vi "TxtToExcel v4.vi"() -> ()   [LabVIEW 2016]
panel:
  out "output array":string[][](array[string])
  out "error out":errorcluster
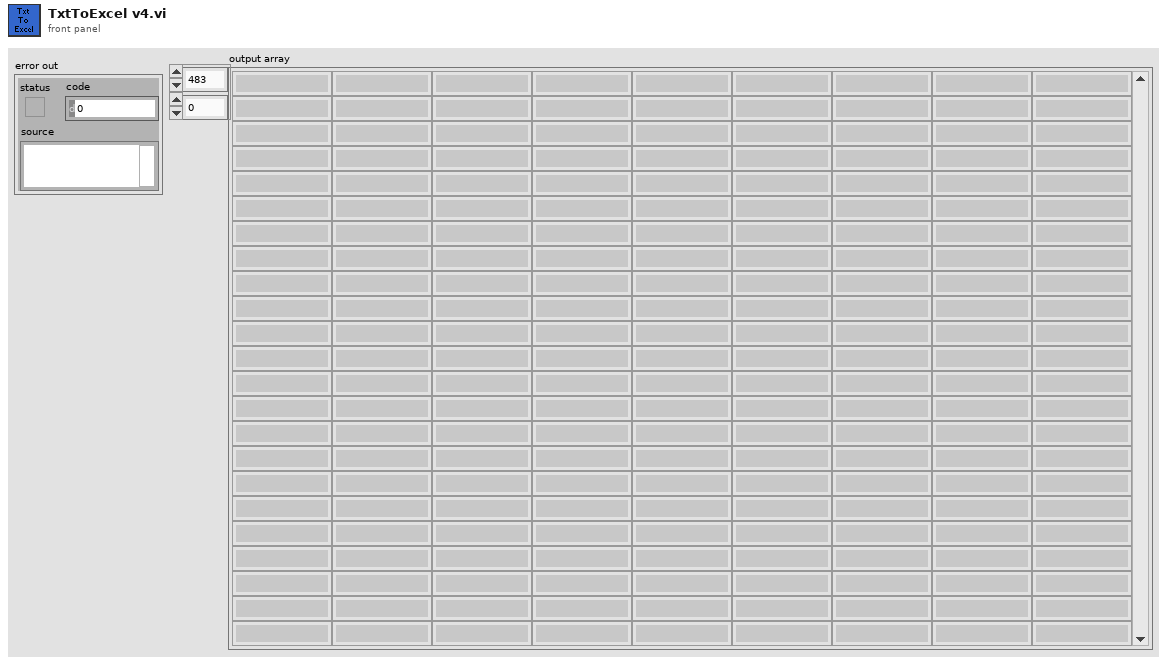
[diagram p1: front panel]
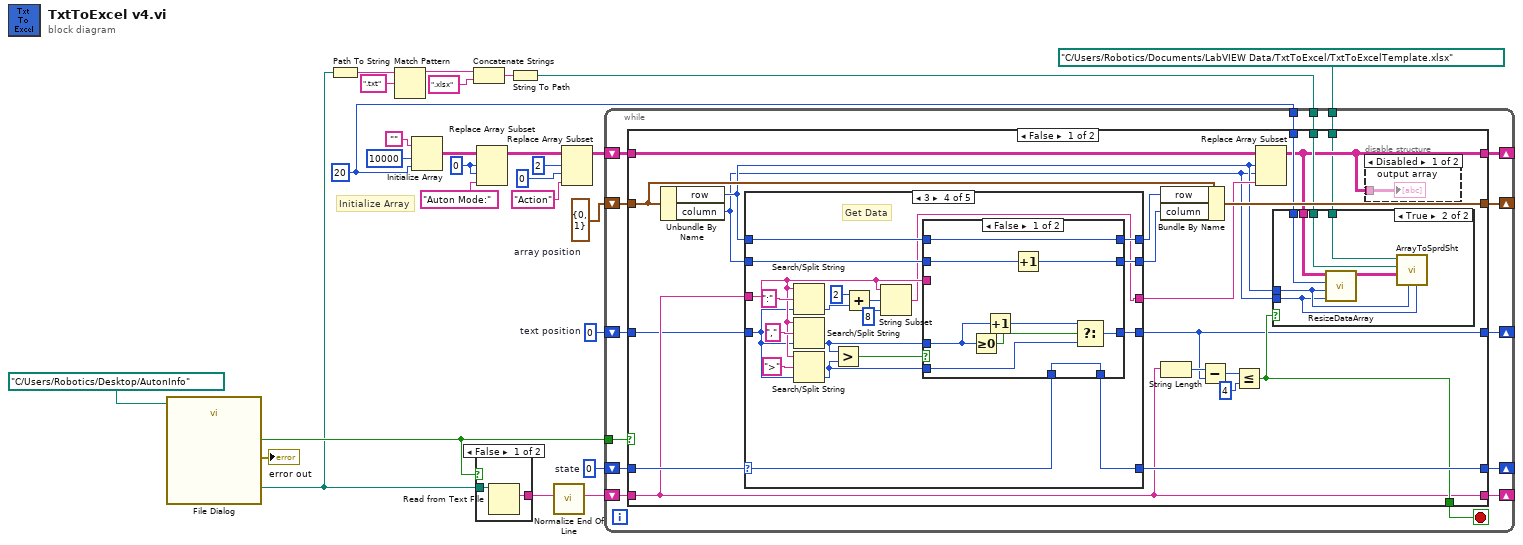
[diagram p0: block diagram]
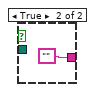
[diagram p2: hidden frame]
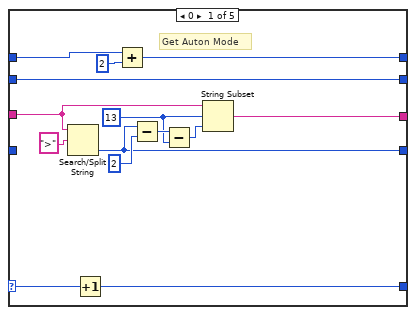
[diagram p5: hidden frame]
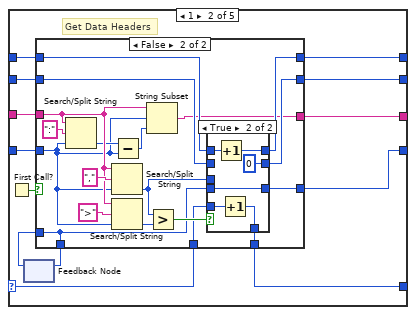
[diagram p6: hidden frame]
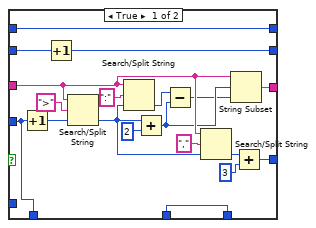
[diagram p7: hidden frame]
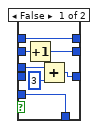
[diagram p8: hidden frame]
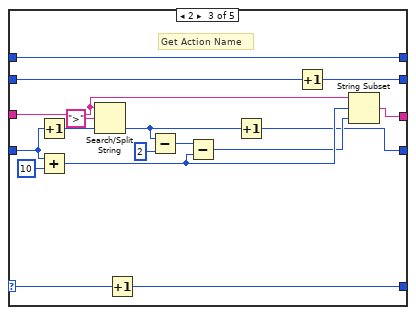
[diagram p9: hidden frame]
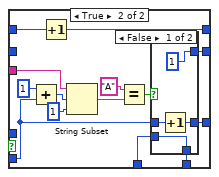
[diagram p10: hidden frame]
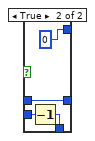
[diagram p11: hidden frame]
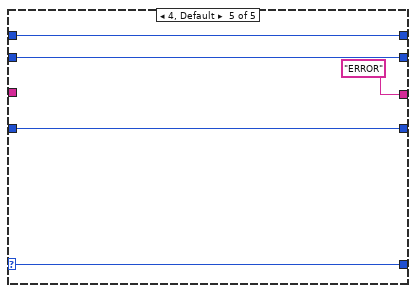
[diagram p12: hidden frame]
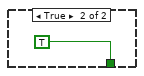
[diagram p13: hidden frame]
diagram:
  w2 = 0  # text position
  w17 = 0 ("index (row)")
  w19 = cluster{"row":i32, "column":i32} {"row"=0, "column"=1}  # array position
  w3 = 20 ("Column Max")
  w24 = 0  # state
  # "Initialize Array"
  n1 = call "File Dialog"("start path"=path "C:/Users/Robotics/Desktop/AutonInfo") -> ("selected path"=w10:path, "cancelled"=w25:bool, "error out"=→"error out":errorcluster)  [unwired: 11 in, 1 out]
  n2 = Path To String(path=w10) -> (string=w9:string)
  n3 = Match Pattern(string=w9, regular expression=".txt") -> (before substring=w5:string)  [unwired: 1 in, 3 out]
  n4 = Initialize Array("", 10000 ("Row Max"), w3) -> (w18:string[][])
  n5 = Concatenate Strings(w5, ".xlsx" ("string")) -> (w7:string)
  n6 = case shown="False" w25 {
    tunnel: w10 -> [w29 _]
    tunnel: [w28 ""] -> w23
    frame False {
      n7 = Read from Text File(file (use dialog)=w29) -> (text=w28:string)  [unwired: 3 in, 3 out]
    }
    frame True {
    }
  }
  n8 = Replace Array Subset(array=w18, new element="Auton Mode:" ("new element/subarray"), index (row)=w17, index (col)=w17) -> (w15:string[][])
  n9 = String To Path(string=w7) -> (path=w6:path)
  n10 = call <vilib>:"Normalize End Of Line.vi"("string in"=w23) -> ("string out"=w22:string)  [unwired: 7 in]
  n11 = Replace Array Subset(array=w15, new element="Action" ("new element/subarray"), index (row)=2, index (col)=0 ("disabled index (col)")) -> (w11:string[][])
  n12 = while {
    tunnel: w25 -> [w45]
    shift-right: [w42] -> _
    shift-left: w24 -> [w43]
    shift-right: [w41] -> _
    shift-left: w22 -> [w40]
    shift-right: [w36] -> _
    shift-left: w11 -> [w38]
    shift-right: [w37] -> _
    shift-left: w19 -> [w39]
    tunnel: w6 -> [w35]
    tunnel: w3 -> [w34]
    shift-right: [w33] -> _
    shift-left: w2 -> [w32]
    tunnel: path "C:/Users/Robotics/Documents/LabVIEW Data/TxtToExcel/TxtToExcelTemplate.xlsx" ("file path (dialog if empty)") -> [w31]
    stop <- w44 stop-if-true
    n13 = case shown="False" w45 {
      tunnel: [w57 TRUE] -> w44
      tunnel: w43 -> [w66 _]
      tunnel: [w65 _] -> w42
      tunnel: [w51 _] -> w41
      tunnel: w40 -> [w51 _]
      tunnel: w39 -> [w62 _]
      tunnel: w38 -> [w61 _]
      tunnel: [w63 _] -> w37
      tunnel: [w52 _] -> w36
      tunnel: w35 -> [w56 _]
      tunnel: w34 -> [w53 _]
      tunnel: [w49 _] -> w33
      tunnel: w32 -> [w47 _]
      tunnel: w31 -> [w46 _]
      frame False {
        n14 = Unbundle By Name(w62) -> ("row"=w55:i32, "column"=w54:i32)
        n15 = case shown="3" w66 {
          selector: w66 -> [w84 w90 w164 w178 w225]
          tunnel: [w87 w101 w169 w172 "ERROR" ("string out")] -> w60
          tunnel: w55 -> [w86 w100 w167 w184 w224]
          tunnel: [w82 w97 w167 w183 w224] -> w59
          tunnel: w54 -> [w75 w99 w168 w187 w223]
          tunnel: [w75 w96 w166 w186 w223] -> w58
          tunnel: [w83 w89 w165 w177 w225] -> w65
          tunnel: w51 -> [w80 w95 w158 w176 _]
          tunnel: [w76 w91 w153 w179 w222] -> w49
          tunnel: w47 -> [_ w93 w160 w175 w222]
          frame 0 {
            w78 = 13 ("y")
            # "Get Auton Mode"
            n16 = Search/Split String(string=w80, search string/char (-)=">") -> (offset of match=w76:i32)  [unwired: 1 in, 2 out]
            n17 = Increment(x=w84) -> (x+1=w83:i32)
            n18 = Add(x=w86, y=2) -> (x+y=w82:i32)
            n19 = Subtract(x=w76, y=2) -> (x-y=w79:i32)
            n20 = Subtract(x=w79, y=w78) -> (x-y=w77:i32)
            n21 = String Subset(string=w80, offset (0)=w78, length (rest)=w77) -> (substring=w87:string)
          }
          frame 1 {
            # "Get Data Headers"
            n22 = First Call?() -> (First Call?: T/F=w98:bool)
            n23 = feedback #1() -> (w92:i32)  [unwired: 1 in]
            n24 = case shown="False" w98 {
              tunnel: [w120 w122] -> w101
              tunnel: w100 -> [w117 w134]
              tunnel: [w117 w133] -> w97
              tunnel: w99 -> [w119 w139]
              tunnel: [w118 w138] -> w96
              tunnel: w95 -> [w113 w131]
              tunnel: [w112 w126] -> w94
              tunnel: w93 -> [w112 w128]
              tunnel: w92 -> [_ w126]
              tunnel: [w103 w123] -> w91
              tunnel: w90 -> [w102 w125]
              tunnel: [w102 w124] -> w89
              frame True {
                n25 = Increment(x=w112) -> (x+1=w111:i32)
                n26 = Increment(x=w119) -> (x+1=w118:i32)
                n27 = Search/Split String(string=w113, search string/char (-)=">", offset (0)=w111) -> (offset of match=w110:i32)  [unwired: 2 out]
                n28 = Search/Split String(string=w113, search string/char (-)=":", offset (0)=w110) -> (offset of match=w108:i32)  [unwired: 2 out]
                n29 = Add(x=w110, y=2 ("offset of match")) -> (x+y=w107:i32)
                n30 = Subtract(x=w108, y=w107) -> (x-y=w106:i32)
                n31 = Search/Split String(string=w113, search string/char (-)=",", offset (0)=w110) -> (offset of match=w104:i32)  [unwired: 2 out]
                n32 = String Subset(string=w113, offset (0)=w107, length (rest)=w106) -> (substring=w120:string)
                n33 = Add(x=w104, y=3 ("offset of match")) -> (x+y=w103:i32)
              }
              frame False {
                n34 = Search/Split String(string=w131, search string/char (-)=":", offset (0)=w128) -> (offset of match=w130:i32)  [unwired: 2 out]
                n35 = Search/Split String(string=w131, search string/char (-)=",", offset (0)=w128) -> (offset of match=w121:i32)  [unwired: 2 out]
                n36 = Search/Split String(string=w131, search string/char (-)=">", offset (0)=w128) -> (offset of match=w135:i32)  [unwired: 2 out]
                n37 = Subtract(x=w130, y=w128) -> (x-y=w129:i32)
                n38 = String Subset(string=w131, offset (0)=w128, length (rest)=w129) -> (substring=w122:string)
                n39 = Greater?(x=w121, y=w135) -> (0:w127:bool)
                n40 = case shown="True" w127 {
                  tunnel: w139 -> [w146 _]
                  tunnel: [w145 0] -> w138
                  tunnel: w134 -> [w144 w151]
                  tunnel: [w144 w150] -> w133
                  tunnel: w126 -> [_ w149]
                  tunnel: [w143 w149] -> w123
                  tunnel: w125 -> [w142 w148]
                  tunnel: [w142 w147] -> w124
                  tunnel: w121 -> [w141 _]
                  frame False {
                    n41 = Increment(x=w146) -> (x+1=w145:i32)
                    n42 = Add(x=w141, y=3 ("x")) -> (x+y=w143:i32)
                  }
                  frame True {
                    n43 = Increment(x=w151) -> (x+1=w150:i32)
                    n44 = Increment(x=w148) -> (x+1=w147:i32)
                  }
                }
              }
            }
            n45 = feedback-in #1(w94) -> ()
          }
          frame 2 {
            # "Get Action Name"
            n46 = Increment(x=w160) -> (x+1=w162:i32)
            n47 = Add(x=w160, y=10) -> (x+y=w156:i32)
            n48 = Search/Split String(string=w158, search string/char (-)=">", offset (0)=w162) -> (offset of match=w154:i32)  [unwired: 2 out]
            n49 = Increment(x=w164) -> (x+1=w165:i32)
            n50 = Subtract(x=w154, y=2) -> (x-y=w157:i32)
            n51 = Subtract(x=w157, y=w156) -> (x-y=w155:i32)
            n52 = Increment(x=w154) -> (x+1=w153:i32)
            n53 = Increment(x=w168) -> (x+1=w166:i32)
            n54 = String Subset(string=w158, offset (0)=w156, length (rest)=w155) -> (substring=w169:string)
          }
          frame 3 {
            # "Get Data"
            n55 = Search/Split String(string=w176, search string/char (-)=":", offset (0)=w175) -> (offset of match=w181:i32)  [unwired: 2 out]
            n56 = Search/Split String(string=w176, search string/char (-)=",", offset (0)=w175) -> (offset of match=w170:i32)  [unwired: 2 out]
            n57 = Search/Split String(string=w176, search string/char (-)=">", offset (0)=w175) -> (offset of match=w171:i32)  [unwired: 2 out]
            n58 = Greater?(x=w170, y=w171) -> (0:w185:bool)
            n59 = Add(x=2 ("y"), y=w181) -> (x+y=w174:i32)
            n60 = String Subset(string=w176, offset (0)=w174, length (rest)=8 ("y")) -> (substring=w172:string)
            n61 = case shown="False" w185 {
              tunnel: w187 -> [w198 _]
              tunnel: [w197 w203] -> w186
              tunnel: w184 -> [w196 w210]
              tunnel: [w196 w209] -> w183
              tunnel: w170 -> [w191 _]
              tunnel: [w194 w199] -> w179
              tunnel: w178 -> [w195 w202]
              tunnel: [w195 w201] -> w177
              tunnel: w176 -> [_ w207]
              tunnel: w171 -> [w190 w200]
              frame False {
                n62 = Greater Or Equal To 0?(x=w191) -> (x >= 0?=w193:bool)
                n63 = Increment(x=w191) -> (x+1=w192:i32)
                n64 = Increment(x=w198) -> (x+1=w197:i32)
                n65 = Select(t=w192, s=w193, f=w190) -> (s? t:f=w194:i32)
              }
              frame True {
                n66 = Add(x=1 ("y"), y=w200) -> (x+y=w205:i32)
                n67 = Increment(x=w210) -> (x+1=w209:i32)
                n68 = String Subset(string=w207, offset (0)=w205, length (rest)=1 ("length (rest)")) -> (substring=w212:string)
                n69 = Equal?(x="A", y=w212) -> (x = y?=w204:bool)
                n70 = case shown="False" w204 {
                  tunnel: [1 ("length (rest)") 0 ("length (rest)")] -> w203
                  tunnel: w202 -> [w213 w219]
                  tunnel: [w213 w218] -> w201
                  tunnel: w200 -> [w216 w217]
                  tunnel: [w215 w217] -> w199
                  frame False {
                    n71 = Increment(x=w216) -> (x+1=w215:i32)
                  }
                  frame True {
                    n72 = Decrement(x=w219) -> (x-1=w218:i32)
                  }
                }
              }
            }
          }
          frame 4, Default {
          }
        }
        n73 = Bundle By Name(cluster=w62, "row"=w59, "column"=w58) -> (w63:cluster{"row":i32, "column":i32})
        n74 = String Length(string=w51) -> (length=w50:i32)
        n75 = Subtract(x=w50, y=w49) -> (x-y=w48:i32)
        n76 = Less Or Equal?(x=w48, y=4) -> (x <= y?=w57:bool)
        n77 = Replace Array Subset(array=w61, new element=w60, index (row)=w55, index (col)=w54) -> (w52:string[][])
        n78 = case shown="True" w57 {
          tunnel: w52 -> [_ w73]
          tunnel: w56 -> [_ w74]
          tunnel: w55 -> [_ w70]
          tunnel: w54 -> [_ w69]
          tunnel: w53 -> [_ w72]
          tunnel: w46 -> [_ w68]
          frame False {
          }
          frame True {
            n79 = call "ResizeDataArray.vi"("Column"=w69, "Row"=w70, "Column Max"=w72, "Input Array"=w73) -> ("Output Array"=w71:string[][])  [unwired: 3 in]
            n80 = call "ArrayToSprdSht.vi"("Column End"=w69, "Row End"=w70, "TextArray"=w71, "report file path"=w74, "template (empty)"=w68) -> ()  [unwired: 7 in]
          }
        }
        n81 = disable-structure shown="Disabled" {
          disable-tunnel: w52 -> [w67 _]
          frame Disabled {
            "output array" <- w67
          }
          frame Enabled {
          }
        }
      }
      frame True {
      }
    }
  }
